vi "Konvolucio MUDS150628 B232EATC Session ClearDTCInformation.vi"   [LabVIEW 2011]
uses:
  <instrlib>/Konvolucio MUDS150628/Konvolucio MUDS150628.lvlib
types:
  T1 = typedef "Konvolucio MUDS150628.lvlib/UdsHandleType.ctl" = cluster{"LogPath":path, "LogEnabled":bool, "isOpen":bool, "LogContent":string, "Adapter":string, "MCanHandle":T2, "TransmittId":u32, "ReceiveId":u32}
  T2 = typedef "Konvolucio MCAN120803.lvlib/MCanHandleType.ctl" = cluster{"MCanAdapter":refnum<k24>}
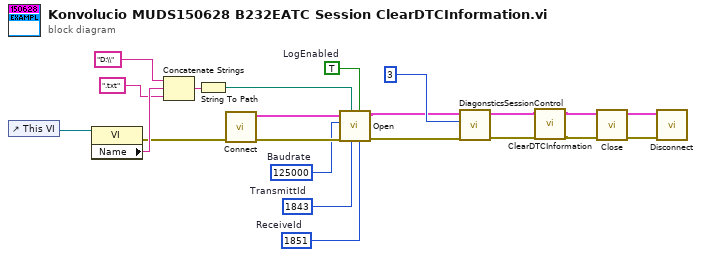
[diagram p0: block diagram]
diagram:
  w9 = TRUE  # LogEnabled
  w8 = u32 125000  # Baudrate
  w5 = u32 1851  # ReceiveId
  w6 = u32 1843  # TransmittId
  n1 = control-ref of="This VI"() -> (w17:refnum<vi>)
  n2 = property class="VI"(reference=w17) -> (error out=w12:errorcluster, "Name"=w15:string)  [unwired: 1 in, 1 out]
  n3 = Concatenate Strings("D:\\" ("VI Name"), w15, ".txt" ("string")) -> (w13:string)
  n4 = String To Path(string=w13) -> (path=w7:path)
  n5 = call <instrlib>:"Connect.vi"("error in"=w12) -> ("error out"=w10:errorcluster, "UdsHandleOut"=w11:T1)  [unwired: 9 in]
  n6 = call <instrlib>:"Open.vi"("ReceiveId"=w5, "LogEnabled"=w9, "TransmittId"=w6, "LogPath"=w7, "error in"=w10, "BaudRate"=w8, "UdsHandleIn"=w11) -> ("error out"=w4:errorcluster, "UdsHandleOut"=w3:T1)  [unwired: 3 in]
  n7 = call <instrlib>:"DiagonsticsSessionControl.vi"("error in"=w4, "Session"=u8 3, "UdsHandleIn"=w3) -> ("error out"=w19:errorcluster, "UdsHandleOut"=w20:T1)  [unwired: 7 in]
  n8 = call <instrlib>:"ClearDTCInformation.vi"("error in"=w19, "UdsHandleIn"=w20) -> ("error out"=w18:errorcluster, "UdsHandleOut"=w21:T1)  [unwired: 8 in]
  n9 = call <instrlib>:"Close.vi"("error in"=w18, "UdsHandleIn"=w21) -> ("error out"=w2:errorcluster, "UdsHandleOut"=w1:T1)  [unwired: 8 in]
  n10 = call <instrlib>:"Disconnect.vi"("error in"=w2, "UdsHandleIn"=w1) -> ()  [unwired: 9 in, 1 out]
